vi "Autotest.vi"(8 "error in (no error)":errorcluster caption="entrée d'erreur (pas d'erreur)", 11 "Class Multimeter Rigol DM3058 en entrée":refnum<class "Class Multimeter Rigol DM3058.lvclass">) -> (0 "error out":errorcluster caption="sortie d'erreur", 2 "Autotest Ok ?":bool, 3 "Class Multimeter Rigol DM3058 en sortie":refnum<class "Class Multimeter Rigol DM3058.lvclass">)   [LabVIEW 2020, in "Library Instrument & Equipement.lvlib" / "Library Multimeter.lvlib" / "Class Multimeter Rigol DM3058.lvclass"]
uses:
  Class Multimeter Rigol DM3058.lvclass
  C:/Users/ngarcin/OneDrive - Altyor/Standard TB/Class/Multimeter/Multimeter (Default)/Class Multimeter (Default).lvclass
  Class Multimeter Rigol DM3058.lvclass/Class Multimeter Rigol DM3058.ctl
  RIGOL DM3058/RIGOL DM3058.lvlib
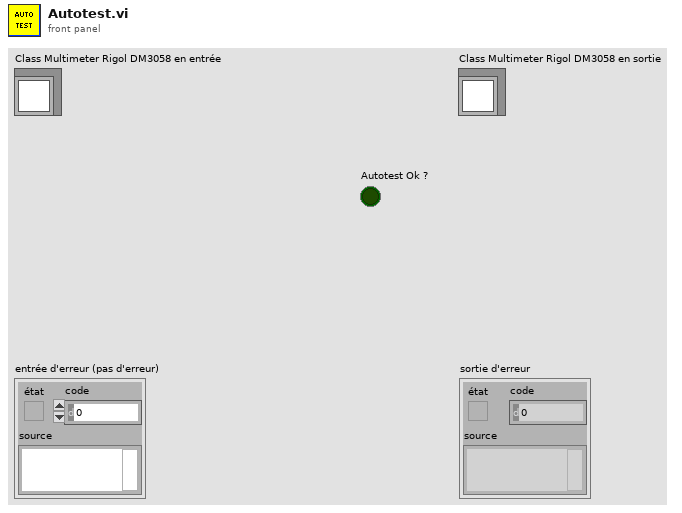
[diagram p1: front panel]
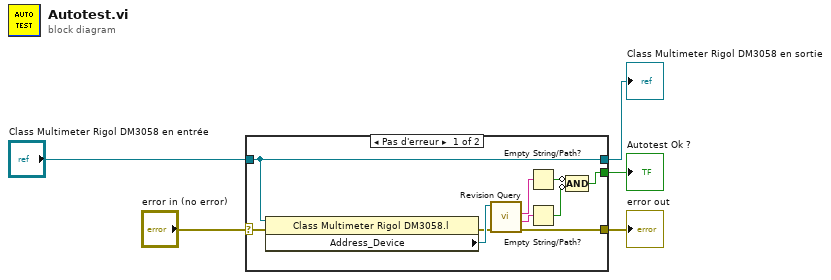
[diagram p0: block diagram]
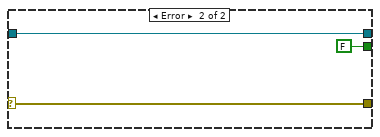
[diagram p2: hidden frame]
diagram:
  n1 = case shown="Pas d'erreur" "error in (no error)" {
    selector: "error in (no error)" -> [w7 w18]
    tunnel: [w15 w18] -> w4
    tunnel: [w9 w17] -> w1
    tunnel: "Class Multimeter Rigol DM3058 en entrée" -> [w9 w17]
    tunnel: [w10 FALSE] -> w5
    frame No Error {
      n2 = property class="Class Multimeter Rigol DM3058.l"(reference=w9, error in=w7) -> (error out=w6:errorcluster, "Address_Device"=w8:refnum<visa-resource-name>)  [unwired: 1 out]
      n3 = call "Revision Query.vi"("error in (no error)"=w6, "VISA resource name"=w8) -> ("error out"=w15:errorcluster, "Instrument Firmware Revision"=w13:string, "Instrument Driver Revision"=w14:string)  [unwired: 6 in, 1 out]
      n4 = Empty String/Path?(string/path=w14) -> (empty?=w12:bool)
      n5 = Empty String/Path?(string/path=w13) -> (empty?=w11:bool)
      n6 = Compound Arithmetic op=AND ("Opérateur arithmétique")(invert w12, invert w11) -> (w10:bool)
    }
    frame Error {
    }
  }
  "error out" <- w4
  "Class Multimeter Rigol DM3058 en sortie" <- w1
  "Autotest Ok ?" <- w5
